vi "Save_to_Project.vi"(8 "error in (no error)":errorcluster, 9 "index":string, 10 "buildObject":T1, 11 "IB_Destination in":refnum<class "IB_Destination.lvclass">) -> (0 "error out":errorcluster, 1 "index out":string, 2 "buildObject out":T1, 3 "IB_Destination out":refnum<class "IB_Destination.lvclass">, 5 "saved?":bool)   [LabVIEW 2020, in "IB_Destination.lvclass"]
uses:
  <vilib>/AppBuilder/IB_Classes/Destination/IB_Destination.lvclass
  <vilib>/AppBuilder/IB_Classes/Destination/IB_Destination.lvclass/IB_Destination.ctl
  <vilib>/AppBuilder/IB_RW_Project/IB_RW_Project_PropBag_Action.ctl
  <vilib>/AppBuilder/IB_RW_Project/IB_RW_Project_Destination_Data.ctl
  <resource>/Framework/Providers/API/ItemRef.ctl
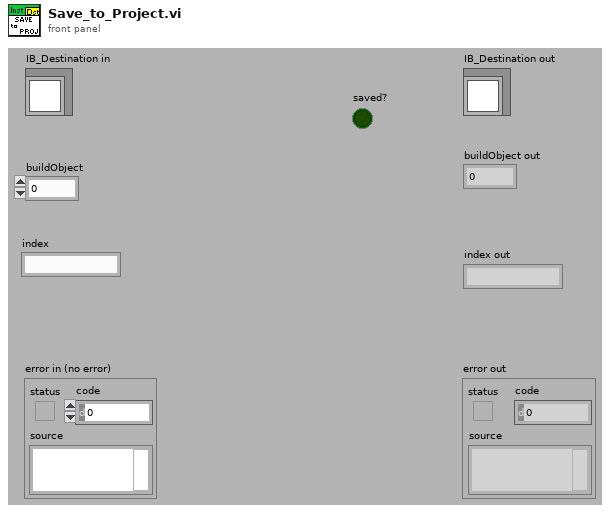
[diagram p1: front panel]
types:
  T1 = typedef "ItemRef.ctl" = u64
  T2 = typedef "IB_RW_Project_PropBag_Action.ctl" = enum16{"read", "write", "clear", "readPrevious", "writePrevious", "clearPrevious"}
  T3 = typedef "IB_RW_Project_Destination_Data.ctl" = cluster{"name":string, "tag":string, "parent":string, "unlock":bool}
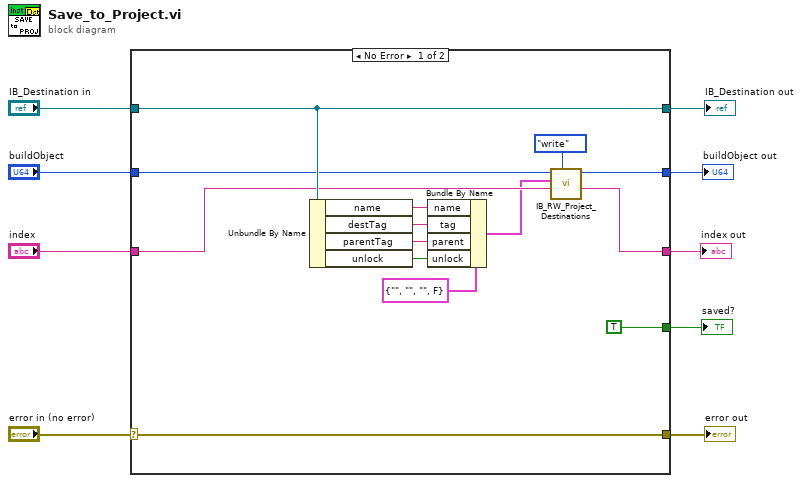
[diagram p0: block diagram]
diagram:
  n1 = case shown="No Error" "error in (no error)" {
    selector: "error in (no error)" -> [w23 w27]
    tunnel: [w23 w27] -> w8
    tunnel: [w20 w26] -> w6
    tunnel: "IB_Destination in" -> [w20 w26]
    tunnel: "buildObject" -> [w18 w25]
    tunnel: "index" -> [w17 w24]
    tunnel: [w12 w25] -> w4
    tunnel: [w11 w24] -> w2
    tunnel: [TRUE _] -> w1
    frame No Error {
      n2 = Unbundle By Name(w20) -> ("name"=w21:string, "destTag"=w15:string, "parentTag"=w14:string, "unlock"=w13:bool)
      n3 = Bundle By Name(cluster=T3 {"name"="", "tag"="", "parent"="", "unlock"=FALSE} ("data in"), "name"=w21, "tag"=w15, "parent"=w14, "unlock"=w13) -> (w16:T3)
      n4 = call <vilib>:"IB_RW_Project_Destinations.vi"("action"=IB_RW_Project_PropBag_Action."write", "index"=w17, "data"=w16, "buildObject"=w18) -> ("index out"=w11:string, "buildObject out"=w12:T1)  [unwired: 4 in, 2 out]
    }
    frame Error {
    }
  }
  "error out" <- w8
  "IB_Destination out" <- w6
  "buildObject out" <- w4
  "index out" <- w2
  "saved?" <- w1
